vi "Get ErrorRemote Event.vi"(8 "error in (no error)":errorcluster, 11 "ErrorHandler in":refnum<class "ErrorHandler.lvclass">) -> (0 "error out":errorcluster, 2 "ErrorRemote Ev":refnum<user-event>, 3 "ErrorHandler out":refnum<class "ErrorHandler.lvclass">)   [LabVIEW 2017, in "ErrorHandler.lvclass"]
doc: "Developed by Kevin Thompson\nkevin@thompsonengineering.net\n\nCopyright 2018\nThompson Engineering, LLC"
uses:
  ErrorHandler.lvclass
  TypeDef/ErrorRemote EventData.ctl
  ErrorHandler.lvclass/ErrorHandler.ctl
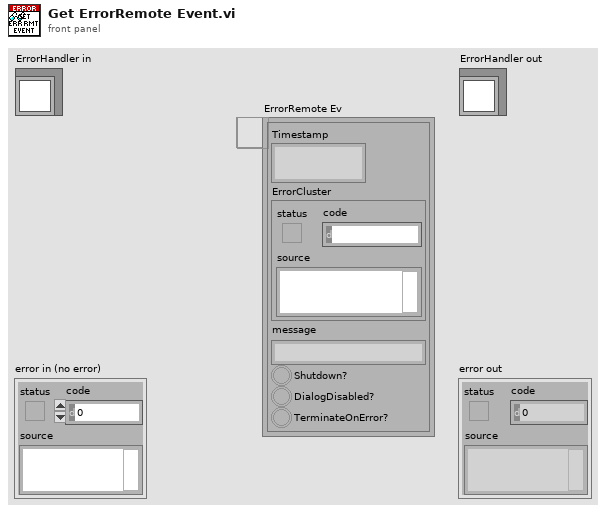
[diagram p1: front panel]
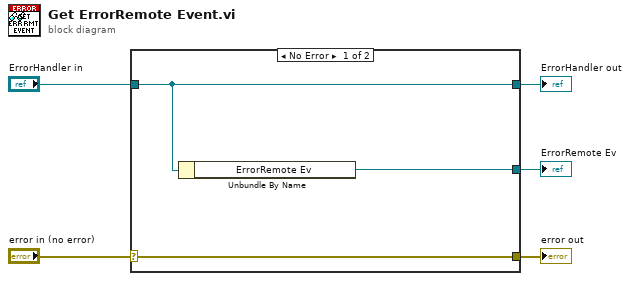
[diagram p0: block diagram]
diagram:
  n1 = case shown="No Error" "error in (no error)" {
    selector: "error in (no error)" -> [w8 w9]
    tunnel: [w8 w9] -> w4
    tunnel: [w7 w10] -> w2
    tunnel: "ErrorHandler in" -> [w7 w10]
    tunnel: [w6 _] -> w1
    frame No Error {
      n2 = Unbundle By Name(w7) -> ("ErrorRemote Ev"=w6:refnum<user-event>)
    }
    frame Error {
    }
  }
  "error out" <- w4
  "ErrorHandler out" <- w2
  "ErrorRemote Ev" <- w1
